vi "Write BMP Data To Buffer.vi"(4 "icon mask data":u8[](array[numeric]), 6 "data":u8[](array[numeric]), 7 "color table":u32[](array[colorbox]), 8 "error in (no error)":errorcluster, 9 "bmp is for icon? (F)":bool, 11 "bmp header":T1) -> (0 "error out":errorcluster, 3 "buffer":string)   [LabVIEW 2020]
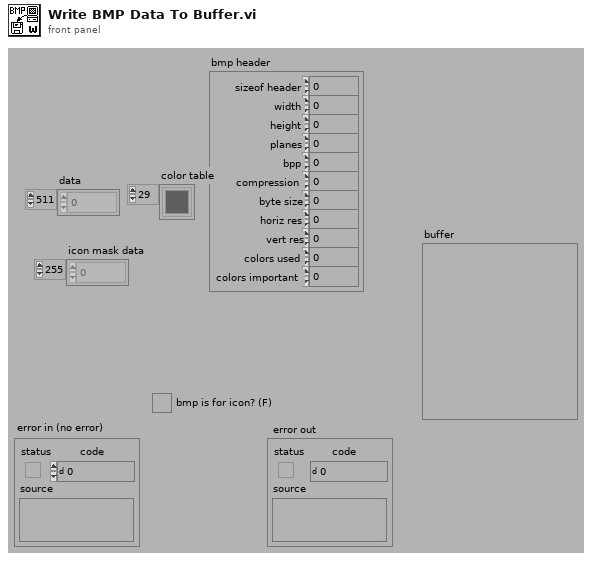
[diagram p1: front panel]
types:
  T1 = cluster{"sizeof header":u32, "width":u32, "height":u32, "planes":u16, "bpp":u16, "compression":u32, "byte size":u32, "horiz res":u32, "vert res":u32, "colors used":u32, "colors important":u32}
  T2 = cluster{"height":u32, "width":u32, "bpp":u16, "padded width":i32}
  T3 = cluster{"height":u32, "width":u32, "bit depth":i32, "padded width":i32}
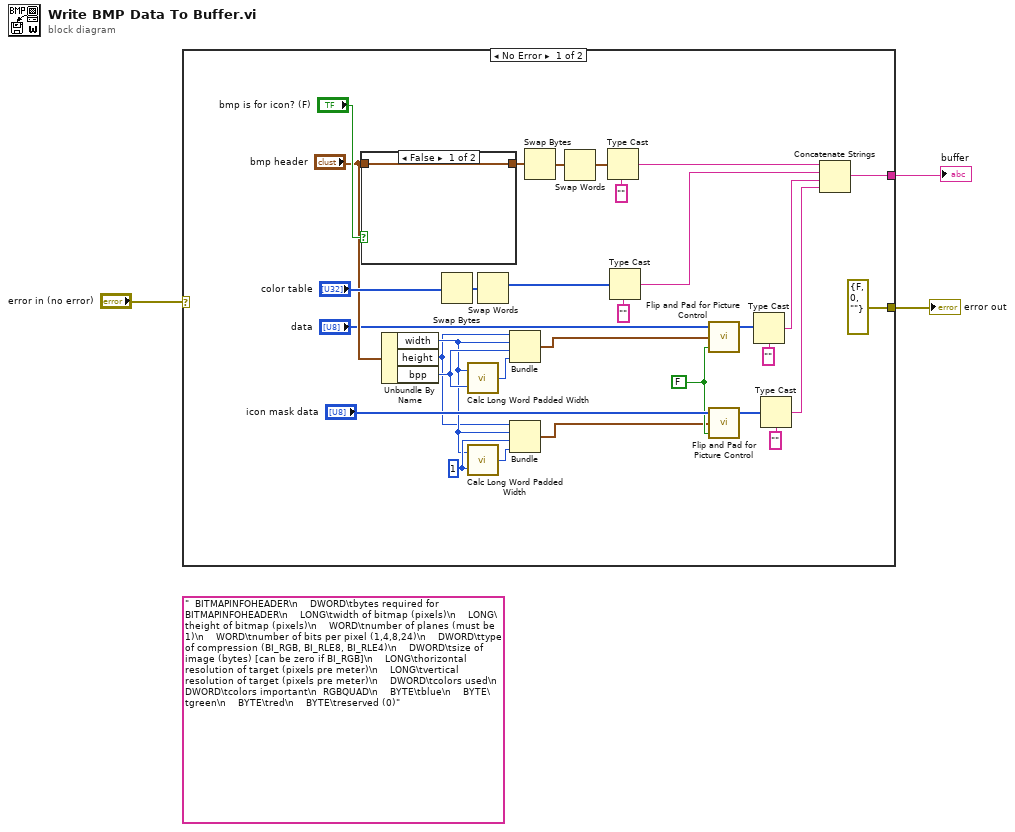
[diagram p0: block diagram]
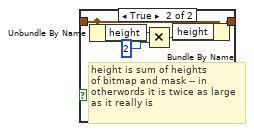
[diagram p2: hidden frame]
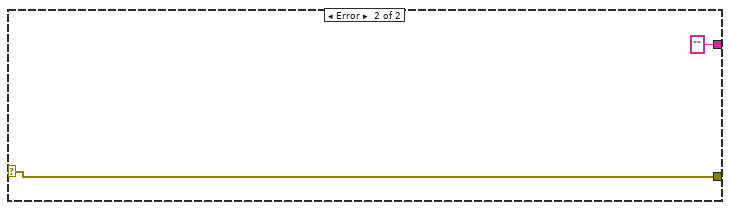
[diagram p3: hidden frame]
diagram:
  (unwired) "  BITMAPINFOHEADER\n    DWORD\tbytes required for BITMAPINFOHEADER\n    LONG\twidth of bitmap (pixels)\n    LONG\theight of bitmap (pixels)\n    WORD\tnumber of planes (must be 1)\n    WORD\tnumber of bits per pixel (1,4,8,24)\n    DWORD\ttype of compression (BI_RGB, BI_RLE8, BI_RLE4)\n    DWORD\tsize of image (bytes) [can be zero if BI_RGB]\n    LONG\thorizontal resolution of target (pixels pre meter)\n    LONG\tvertical resolution of target (pixels pre meter)\n    DWORD\tcolors used\n    DWORD\tcolors important\n  RGBQUAD\n    BYTE\tblue\n    BYTE\tgreen\n    BYTE\tred\n    BYTE\treserved (0)"
  n1 = case shown="No Error" "error in (no error)" {
    selector: "error in (no error)" -> [_ w42]
    tunnel: [w18 ""] -> w3
    tunnel: [errorcluster {"status"=FALSE, "code"=0, "source"=""} ("error IO") w42] -> w1
    frame No Error {
      w7 = 1 ("bit depth")
      w10 = FALSE ("bmp to LV? (T)")
      n2 = case shown="False" "bmp is for icon? (F)" {
        tunnel: "bmp header" -> [w35 w40]
        tunnel: [w35 w39] -> w16
        frame False {
        }
        frame True {
          # "height is sum of heights\nof bitmap and mask -- in\notherwords it is twice as large\nas it really is"
          n3 = Unbundle By Name(w40) -> ("height"=w38:u32)
          n4 = Multiply(x=w38, y=u8 2) -> (x*y=w37:u32)
          n5 = Bundle By Name(cluster=w40, "height"=w37) -> (w39:T1)
        }
      }
      n6 = Unbundle By Name("bmp header") -> ("width"=w6:u32, "height"=w5:u32, "bpp"=w25:u16)
      n7 = Swap Bytes(anything="color table") -> (byte swapped=w30:u32[])
      n8 = call "Calc Long Word Padded Width.vi"("bit depth"=w25, "width"=w6) -> ("padded width"=w26:i32)
      n9 = call "Calc Long Word Padded Width.vi"("bit depth"=w7, "width"=w6) -> ("padded width"=w9:i32)
      n10 = Swap Words(1:w30) -> (0:w27:u32[])
      n11 = Bundle("height"=w5, "width"=w6, "bpp"=w25, "padded width"=w26) -> (w17:T2)  [unwired: 1 in]
      n12 = Bundle("height"=w5, "width"=w6, "bit depth"=w7, "padded width"=w9) -> (w8:T3)  [unwired: 1 in]
      n13 = Swap Bytes(anything=w16) -> (byte swapped=w33:T1)
      n14 = Swap Words(1:w33) -> (0:w32:T1)
      n15 = Type Cast(type="", x=w32) -> (*(type *) &x=w22:string)
      n16 = Type Cast(type="", x=w27) -> (*(type *) &x=w21:string)
      n17 = call "Flip and Pad for Picture Control.vi"("bmp to LV? (T)"=w10, "bitmap info"=w17, "BMP bitmap"="data") -> ("picture bitmap"=w14:u8[])  [unwired: 2 in]
      n18 = call "Flip and Pad for Picture Control.vi"("bmp to LV? (T)"=w10, "bitmap info"=w8, "BMP bitmap"="icon mask data") -> ("picture bitmap"=w12:u8[])  [unwired: 2 in]
      n19 = Type Cast(type="", x=w14) -> (*(type *) &x=w20:string)
      n20 = Type Cast(type="", x=w12) -> (*(type *) &x=w19:string)
      n21 = Concatenate Strings(w22, w21, w20, w19) -> (w18:string)
    }
    frame Error {
    }
  }
  "error out" <- w1
  "buffer" <- w3
